vi "Set I1 (SubVI).vi"(11 "Current X":string) -> (3 "String instruction":string)   [LabVIEW 2018]
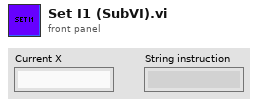
[diagram p1: front panel]
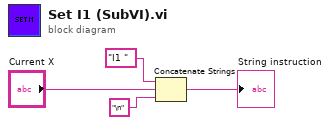
[diagram p0: block diagram]
diagram:
  n1 = Concatenate Strings("I1 ", "Current X", "\n") -> (→"String instruction":string)
